vi "_LaunchHelp.vi"(4 "error in (no error)":errorcluster, 6 "CHM or HLP filename (lvdialog.chm)":string="lvdialog.chm", 7 "HTML filename":string) -> (0 "error out":errorcluster)   [LabVIEW 2021]
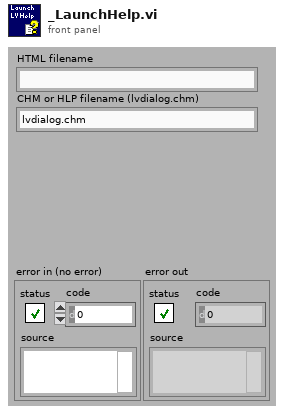
[diagram p1: front panel]
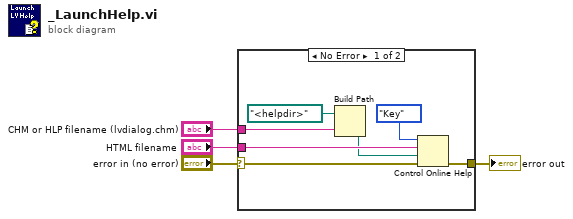
[diagram p0: block diagram]
diagram:
  n1 = case shown="No Error" "error in (no error)" {
    selector: "error in (no error)" -> [w6 w12]
    tunnel: "HTML filename" -> [w10 _]
    tunnel: "CHM or HLP filename (lvdialog.chm)" -> [w8 _]
    tunnel: [w5 w12] -> w2
    frame No Error {
      n2 = Build Path(base path=path "<helpdir>", name or relative path=w8) -> (appended path=w7:path)
      n3 = Control Online Help(1:w6, 2:w7, 3:w10, 4:enum16{"Contents", "Key", "Close"}."Key" ("Operation")) -> (0:w5:errorcluster)
    }
    frame Error {
    }
  }
  "error out" <- w2
